vi "Init.vi"(8 "Error In":errorcluster) -> (0 "Error Out":errorcluster, 3 "Message Queues":T1)   [LabVIEW 2017, in "Client.lvlib" / "CommsFrameWork.lvlib"]
uses:
  CommsFrameWork.lvlib
  ClientErrorHandler.lvlib
  CommsServer.lvlib
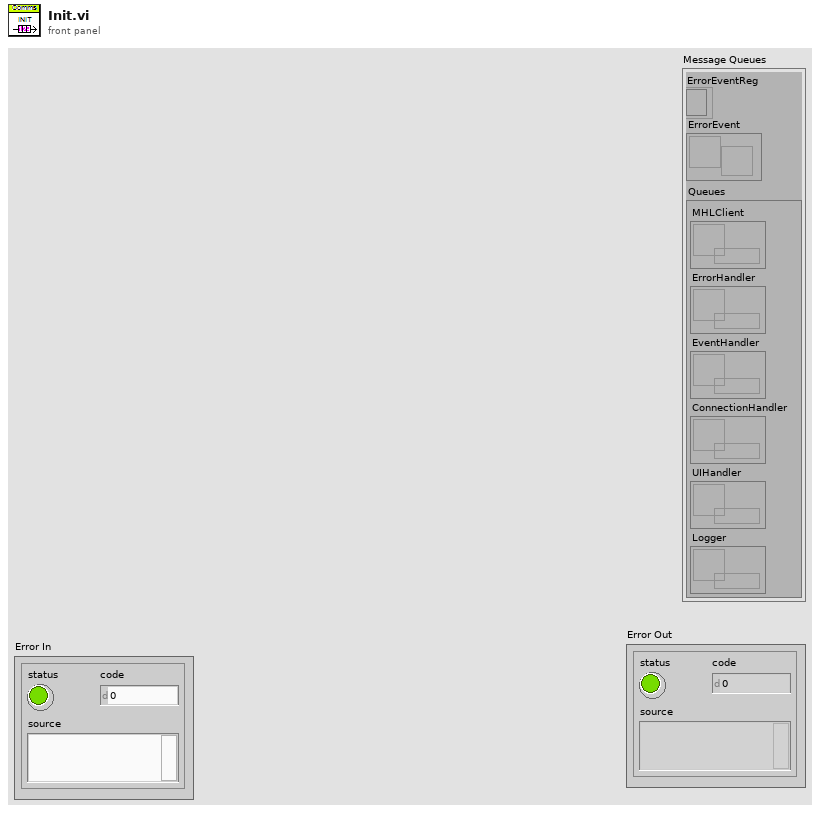
[diagram p1: front panel]
types:
  T1 = cluster{"ErrorEventReg":refnum<event-registration>, "ErrorEvent":refnum<user-event>, "Queues":cluster{"MHLClient":refnum<queue>, "ErrorHandler":refnum<queue>, "EventHandler":refnum<queue>, "ConnectionHandler":refnum<queue>, "UIHandler":refnum<queue>, "Logger":refnum<queue>}}
  T2 = cluster{"Connection Data":cluster{"IP":string, "Port":string, "ClientName":string}}
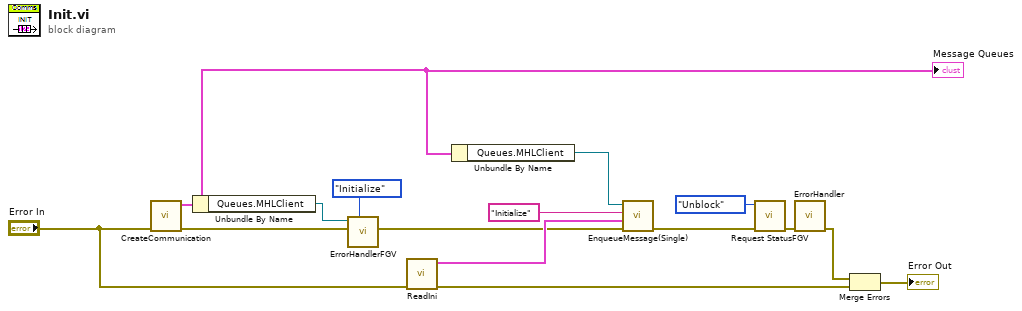
[diagram p0: block diagram]
diagram:
  n1 = call "CreateCommunication.vi"("error in (no error)"="Error In") -> ("error out"=w5:errorcluster, "Message Queues"=w14:T1)  [unwired: 9 in]
  "Message Queues" <- w14
  n2 = Unbundle By Name(w14) -> ("Queues.MHLClient"=w6:refnum<queue>)
  n3 = call "ErrorHandlerFGV.vi"("Command(CheckErrors)"=enum16{"Initialize", "CheckErrors"}."Initialize", "Error In"=w5, "MHL"=w6) -> ("Error Out"=w4:errorcluster)  [unwired: 8 in]
  n4 = call "ReadIni.vi"("Error In"="Error In") -> ("Error Out"=w10:errorcluster, "InternalData"=w11:T2)  [unwired: 9 in]
  n5 = Unbundle By Name(w14) -> ("Queues.MHLClient"=w15:refnum<queue>)
  n6 = call "EnqueueMessage(Single).vi"("error in (no error)"=w4, "Message Data"=w11, "Message"="Initialize", "Message Queue"=w15) -> ("error out"=w2:errorcluster)  [unwired: 6 in, 1 out]
  n7 = call "Request StatusFGV.vi"("Error In"=w2, "Command"=enum16{"Block", "Unblock", "Check Status"}."Unblock") -> ("Error Out"=w1:errorcluster)  [unwired: 8 in, 1 out]
  n8 = call "ErrorHandler.vi"("error in (no error)"=w1) -> ("error out"=w8:errorcluster)  [unwired: 10 in]
  n9 = Merge Errors(w8, w10) -> (→"Error Out":errorcluster)
